vi "day 2 task 2.vi"() -> ()   [LabVIEW 2019]
panel:
  out "size(s)":i32
  out "sum":i32
  out "round scores":i32[](array[numeric])
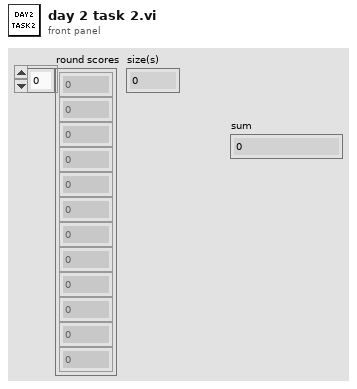
[diagram p1: front panel]
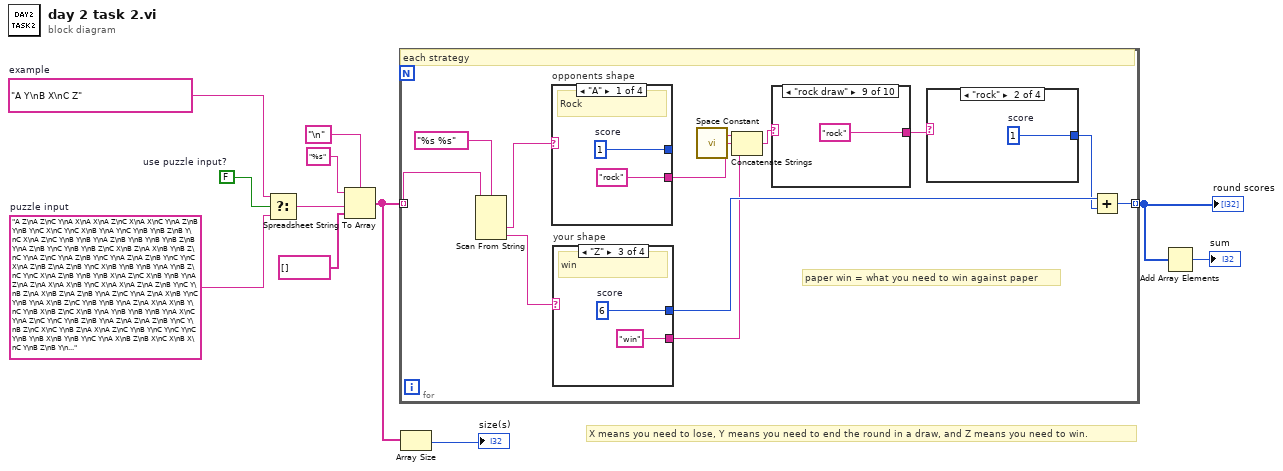
[diagram p0: block diagram]
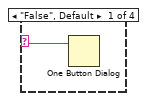
[diagram p2: hidden frame]
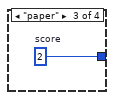
[diagram p3: hidden frame]
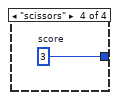
[diagram p4: hidden frame]
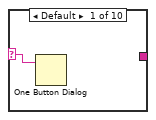
[diagram p5: hidden frame]
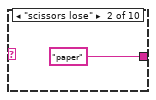
[diagram p6: hidden frame]
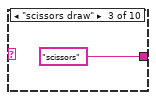
[diagram p7: hidden frame]
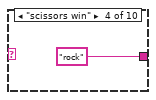
[diagram p8: hidden frame]
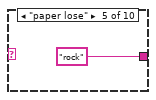
[diagram p9: hidden frame]
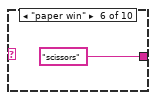
[diagram p10: hidden frame]
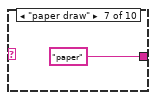
[diagram p11: hidden frame]
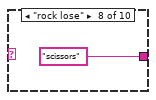
[diagram p12: hidden frame]
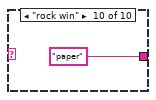
[diagram p13: hidden frame]
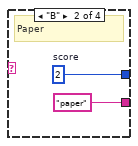
[diagram p14: hidden frame]
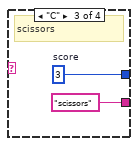
[diagram p15: hidden frame]
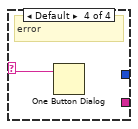
[diagram p16: hidden frame]
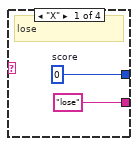
[diagram p17: hidden frame]
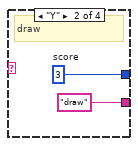
[diagram p18: hidden frame]
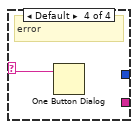
[diagram p19: hidden frame]
diagram:
  w6 = FALSE  # use puzzle input?
  w7 = "A Z\nA Z\nC Y\nA X\nA X\nA Z\nC X\nA X\nC Y\nA Z\nB Y\nB Y\nC X\nC Y\nC X\nB Y\nA Y\nC Y\nB Y\nB Z\nB Y\nC X\nA Z\nC Y\nB Y\nB Y\nA Z\nB Y\nB Y\nB Y\nB Z\nB Y\nA Z\nB Y\nC Y\nB Y\nB Z\nC X\nB Z\nA X\nB Y\nB Z\nC Y\nA Z\nC Y\nA Z\nB Y\nC Y\nA Z\nA Z\nB Y\nC Y\nC X\nA Z\nB Z\nA Z\nB Y\nC X\nB Y\nB Y\nB Y\nA Y\nB Z\nC Y\nC X\nA Z\nB Y\nB Y\nB X\nA Z\nC X\nB Y\nB Y\nA Z\nA Z\nA X\nA X\nB Y\nC X\nA X\nA Z\nA Z\nB Y\nC Y\nB Z\nA X\nB Z\nA Z\nB Y\nA Z\nC Y\nA Z\nA X\nB Y\nC Y\nB Y\nA X\nB Z\nC Y\nB Y\nB Y\nA Z\nA X\nA X\nB Y\nC Y\nB X\nB Z\nC X\nB Y\nA Y\nB Y\nB Y\nB Y\nA X\nC Y\nA Z\nC Y\nC Y\nB Z\nB Y\nA Z\nA Z\nA Z\nB Y\nC Y\nB Z\nC X\nC Y\nB Z\nA X\nA Z\nC Y\nB Y\nC Y\nC Y\nC Y\nB Y\nB X\nB Y\nB Y\nC Y\nA X\nB Z\nB X\nC X\nB X\nC Y\nB Z\nB Y\nA X\nC Y\nC Y\nC X\nB Z\nB Y\nA Y\nB Z\nA Z\nB Y\nB Y\nB Z\nB Z\nC Y\nA Z\nA X\nA X\nC Y\nB Y\nA Z\nB Z\nA X\nA Z\nB Z\nC Y\nC Z\nA X\nA Y\nB Y\nC Y\nB Y\nC Y\nB Z\nB Y\nA Z\nC Y\nB Z\nB Y\nA Z\nA Y\nB Y\nB Y\nC Y\nA Z\nC Y\nB Y\nB Y\nA X\nA Z\nA Z\nB Y\nB Y\nB Z\nC Y\nC X\nB Z\nA Y\nB Z\nA X\nC X\nA Y\nB Z\nB Z\nA X\nC X\nC X\nA Z\nC Y\nA X\nA X\nC X\nA X\nB Z\nC Z\nB Z\nB Y\nB Y\nA Z\nA Z\nB Y\nA Z\nC Y\nC X\nB Y\nA X\nA X\nB Z\nC Y\nC Y\nA X\nB Z\nA X\nC X\nC X\nB Z\nC X\nB Z\nA X\nA Y\nA X\nA Z\nA X\nB Y\nC Y\nA X\nC Y\nA Z\nB Z\nA Z\nC Y\nA X\nA Z\nB Y\nA Z\nB Z\nB Z\nA Z\nB Z\nA X\nB Y\nB Z\nC X\nB Y\nB Y\nB Y\nB Y\nA X\nB Z\nB Z\nA Z\nA Z\nC Y\nB Y\nC X\nA X\nB Y\nB Y\nC X\nB Y\nA X\nC Y\nA Z\nB Y\nA Y\nB Z\nB Y\nA Z\nA X\nB Z\nC Y\nA Z\nC Y\nC X\nB Y\nB Z\nC X\nA Y\nB Z\nA Y\nB Z\nB Z\nB Y\nB Z\nC X\nB Y\nA X\nB Z\nA Z\nB Y\nA Z\nC Y\nC Y\nC X\nC X\nA X\nC X\nA X\nA X\nB Z\nB Y\nB Y\nB Y\nB Y\nC X\nC X\nA Z\nA Z\nC X\nC X\nC Y\nC Y\nC Y\nB Y\nA Z\nC Y\nB Z\nB Z\nB Y\nC X\nC X\nC Y\nC Y\nC X\nB Z\nB Z\nB Y\nC Y\nB Y\nA Z\nC Y\nA X\nB Y\nC Y\nC Y\nC Y\nB Y\nA Z\nB Y\nA X\nB Z\nC X\nA Z\nC X\nA Z\nB Z\nC Y\nC Y\nC Y\nC X\nB Z\nC X\nB Y\nB Z\nC X\nB X\nA Z\nB Z\nB Y\nC Y\nB Z\nC Y\nA X\nB Z\nC Y\nC Y\nB Z\nB Y\nC Y\nB Z\nC Y\nA Z\nC X\nC X\nC Y\nA Z\nC Z\nC Y\nB Y\nC Y\nB Y\nB Y\nB Z\nC X\nC X\nB Z\nB Z\nB Z\nA Z\nB Y\nB Y\nA X\nB Y\nC Y\nB Y\nC X\nC X\nB Y\nB Y\nA Y\nB Z\nB Y\nB Y\nC Y\nA Z\nC X\nA Y\nB Y\nB Z\nB Y\nA Y\nC Y\nA Y\nA Z\nB Y\nA Z\nC Y\nC Y\nB Y\nA Z\nB Y\nB Y\nA Z\nB Z\nB Y\nC X\nC Y\nB Z\nB Y\nB Y\nA Z\nC Z\nA Z\nA X\nC X\nB Z\nB Z\nC X\nC Y\nB Y\nB X\nA X\nC Y\nB Z\nB Y\nC X\nB Y\nA Z\nA Z\nA X\nC Y\nB Z\nB Y\nC X\nC X\nB Y\nA Z\nC Z\nB Y\nA Z\nC Y\nB Y\nC X\nA Z\nA Z\nA X\nC X\nA X\nC X\nC X\nA Z\nC X\nB Y\nA Z\nB Y\nB Y\nC Y\nC X\nA Z\nB Z\nB Y\nB Y\nA Y\nA Z\nB Y\nA Z\nB Z\nB Y\nC Y\nA Z\nB Y\nB Y\nB Y\nC Y\nC X\nA X\nA Z\nB Z\nB Y\nC Y\nB Z\nC X\nB Y\nC X\nA Z\nB Y\nB X\nB Y\nA Y\nA X\nA X\nC X\nC X\nB Y\nB X\nC Y\nA Z\nB Z\nC Y\nC Y\nB Y\nA Z\nC X\nA Z\nC Y\nB Z\nB X\nC X\nB X\nC X\nB Y\nC Y\nC Y\nB Z\nB Y\nB Z\nB Z\nA Z\nB Y\nA Y\nB Z\nC X\nC Y\nC X\nA Z\nB Z\nC Y\nB Y\nB Z\nC X\nB Y\nA Y\nA X\nA X\nC Y\nB X\nC X\nB Z\nA Z\nA Y\nB Z\nC X\nC X\nB Y\nA X\nB Z\nC Y\nB X\nB Z\nC Y\nB Y\nC Y\nB Z\nB Y\nB Z\nB Y\nC X\nB Y\nC X\nB Z\nB Z\nC X\nB Z\nA X\nB X\nB Y\nA X\nB Z\nC X\nB Z\nB Y\nB Y\nC X\nA Y\nB Z\nB Z\nB Y\nB Y\nB Z\nC Y\nB Z\nC Y\nC X\nA Z\nC X\nA X\nC Y\nB Y\nC X\nA Z\nB Y\nA Z\nA Z\nB X\nC Y\nB Z\nC Y\nB Y\nB Z\nA X\nB Z\nA X\nC X\nB Z\nB Y\nC X\nC Y\nC Y\nB X\nC X\nC X\nB Z\nC Y\nB Z\nB Y\nB Z\nC Y\nB Y\nC Y\nC X\nB Y\nB Y\nB Z\nA Z\nC X\nA Z\nB Y\nB Z\nA Z\nC Y\nA Z\nB Y\nA Z\nA Z\nC Y\nA Y\nB Y\nA Y\nC X\nB Y\nC X\nB Z\nC Y\nA Z\nC X\nC X\nB Z\nC Z\nC Z\nB Y\nB Y\nC Y\nC Y\nA Z\nC Y\nC Y\nC Y\nA Z\nB Z\nC Y\nB Y\nC Y\nC X\nC X\nB X\nB Y\nC Y\nA Y\nB Y\nB Z\nB Y\nA Y\nB Y\nB X\nC X\nC Z\nC Y\nC Y\nC Y\nB Z\nB X\nC Y\nB Z\nC X\nC Y\nA Z\nA Y\nB Y\nC X\nA Z\nB Y\nC Y\nB Z\nA Z\nA Z\nB Y\nA Z\nC Y\nA X\nC Y\nB Z\nB Z\nB Z\nB Y\nB Y\nA Z\nA Z\nB Y\nC X\nA Z\nC Y\nB Y\nA Z\nC Y\nA Z\nB Z\nB Z\nA Y\nB Y\nB Y\nB Z\nC Z\nB Y\nB X\nB Y\nC X\nB Z\nC Y\nB Z\nA Y\nB Z\nA Z\nA X\nA Z\nC X\nC X\nB Y\nC X\nC Y\nA Z\nB Z\nB Y\nA Z\nB Z\nB Z\nB Z\nC Y\nB Y\nA X\nC Y\nC Y\nC X\nA X\nC Y\nB Y\nC X\nB Z\nA Y\nB X\nB Y\nA Z\nB Y\nB Y\nB Y\nB Z\nC X\nB Z\nB Z\nC X\nB Y\nA Y\nB Y\nC Y\nA Z\nC Z\nB Y\nB Z\nB Z\nC Y\nA Z\nC Y\nC X\nC Y\nB Y\nA X\nA X\nB Z\nC Y\nB Z\nB Y\nA Y\nC X\nA Z\nB Z\nC Y\nC Z\nC X\nB Y\nC X\nA Y\nA Y\nB Z\nC X\nB X\nC X\nB Y\nB Z\nB Z\nB Y\nC Y\nB Y\nB Y\nA Z\nB Z\nB Y\nC X\nB Z\nB Y\nB Y\nC Y\nC Z\nC X\nB Y\nA X\nC Y\nC X\nB Z\nC Y\nA X\nB Y\nA Y\nB Y\nC X\nC Y\nC X\nA X\nB Z\nC X\nB Y\nA Z\nC X\nB Y\nA Z\nB Y\nB Y\nB Y\nA Z\nA X\nC X\nC Y\nC Y\nB Y\nB Y\nB Z\nA Y\nC X\nC X\nB Y\nB Y\nB Z\nA X\nC X\nC X\nB X\nA X\nB Z\nB Y\nC X\nA X\nB Y\nC Y\nA X\nB Y\nC X\nB Z\nC Z\nB X\nC Y\nB Y\nC Y\nA Z\nC Y\nB Z\nC X\nB Z\nC X\nC Y\nC X\nC Y\nC Z\nC X\nC X\nB Y\nC Y\nC X\nC X\nB Z\nB Z\nA X\nC Y\nC Z\nB Y\nC Z\nC Y\nC X\nC X\nB Y\nC Y\nA Y\nB Y\nA Y\nB Y\nB Y\nB Y\nC Y\nC Z\nB Y\nC X\nC X\nB Z\nB Y\nB Z\nC Y\nB Z\nC X\nB Z\nB Y\nB Y\nA Z\nA X\nB X\nA X\nC X\nC Y\nB Y\nA X\nB Z\nB Y\nB Y\nA X\nC X\nC X\nB Y\nB Y\nC Y\nC Y\nB Z\nB Y\nB Y\nB Y\nC Y\nA X\nB Y\nC Y\nB Z\nB Y\nB Y\nB Z\nB Y\nB Y\nB Z\nB Y\nB Y\nC Y\nA Z\nB Z\nA Y\nB Y\nC Y\nB Z\nB Y\nB Y\nC X\nA X\nC Z\nC X\nB Y\nB Z\nC Y\nC X\nB Z\nA Z\nA Z\nC Y\nA Z\nB Y\nB Y\nB Z\nB Y\nC Y\nB Z\nC Y\nB Z\nB Z\nB Y\nC X\nB Y\nB Z\nA X\nC X\nC X\nB Z\nB Z\nC X\nB Y\nA Z\nB Y\nB Z\nC Y\nB Y\nA Z\nB Z\nB Y\nB Y\nB Y\nC X\nC Y\nA Z\nB Y\nB Y\nA Z\nA Z\nA Z\nA X\nB X\nA Z\nC Y\nC X\nA X\nB Z\nA X\nC X\nB Z\nB Y\nB Y\nC X\nA Z\nC Y\nC X\nA Y\nC X\nA Z\nB Z\nB Z\nB Y\nC Y\nB Z\nA Z\nA Z\nC Y\nB Y\nB Z\nA Z\nA Z\nB Z\nB Y\nA Z\nC Y\nA Z\nA Z\nB Y\nB Z\nB Z\nA X\nA X\nB Y\nB Z\nB Z\nC X\nB Z\nC Z\nB Y\nB Y\nB Y\nB Z\nA X\nA Z\nB Y\nA X\nB Y\nB Y\nC X\nC X\nC Y\nC Y\nA Z\nA X\nB Y\nA Z\nB Z\nB Y\nC X\nB Y\nB X\nC X\nA X\nA Z\nC Y\nC X\nC Y\nB Y\nB Y\nA X\nA Y\nB Y\nA Y\nC Y\nC X\nB Y\nB Y\nB Z\nC X\nC X\nB Y\nC X\nB Z\nC Y\nA X\nA Z\nA Z\nB Y\nA Y\nC Y\nC X\nC Y\nC Y\nB Y\nB Y\nA Z\nC X\nA X\nB Y\nB Y\nB Y\nB Z\nA Z\nB Y\nB Y\nA Z\nB Y\nA Z\nC X\nB Z\nC Y\nB Y\nB Y\nA X\nB Y\nA X\nB Y\nB Z\nC X\nB Z\nB Y\nC X\nC Y\nC Y\nA X\nA X\nB Z\nB Z\nB Y\nC X\nA Z\nC Y\nC Y\nC Y\nB Z\nB Z\nB Y\nA Z\nC Y\nA X\nA Z\nC Y\nB Z\nB Y\nB Y\nA Z\nB Y\nA Z\nC X\nA X\nB Z\nB Y\nB Y\nB Z\nA Z\nC X\nB Y\nC X\nB Z\nC X\nA Z\nB Y\nA Z\nA Z\nB Y\nC Y\nC X\nC Y\nA X\nC Y\nB Y\nB Z\nC X\nC Y\nA X\nB Z\nB Y\nC Y\nA X\nB Z\nA Y\nB Z\nB Y\nB Z\nA X\nA Z\nA X\nB Z\nC Y\nB Y\nA Y\nB Z\nA Z\nC Y\nC X\nB Z\nB Y\nC Y\nB Z\nC X\nC Y\nA X\nB Z\nB Z\nB Z\nB Z\nB Y\nC X\nB Y\nC X\nA Z\nA Z\nC Y\nA Y\nB Y\nC X\nA Z\nB Z\nC X\nC X\nA X\nB Y\nC X\nA Z\nB Y\nB Y\nB Y\nB Y\nC X\nC Y\nC Y\nB Y\nA Z\nB Y\nB Z\nB Z\nB Y\nA X\nB Z\nB Z\nC X\nC X\nC Y\nB Y\nC Y\nB Y\nB Y\nB Z\nB X\nC X\nC Y\nA Z\nB Z\nB Y\nA X\nB Z\nA Z\nB Z\nB Y\nB Y\nA Z\nC Y\nB Y\nC Y\nB Z\nB Y\nC X\nB Z\nB Z\nC Y\nC Y\nB Y\nC Y\nC X\nB X\nB Y\nC Y\nB Y\nB X\nC X\nB Y\nA Y\nA Z\nA Y\nB Z\nA Z\nA Z\nA Z\nB Y\nA Z\nA Z\nC Y\nB Z\nA Z\nA X\nB Y\nC Y\nC X\nC X\nA Z\nB Z\nB X\nB Z\nC X\nB Z\nC Y\nC X\nC Z\nC X\nB Z\nB Z\nB Z\nB Z\nA Z\nA Z\nC Y\nC Z\nC Y\nA X\nB Y\nB Y\nB Y\nA Z\nA Z\nB Z\nC Y\nC X\nB Y\nC X\nB Z\nB Y\nB Y\nB Y\nB Y\nB Y\nB X\nA Z\nA X\nA Y\nC X\nB Z\nB Y\nB Z\nC Y\nA Z\nB Z\nB Z\nC Y\nB Z\nB Z\nC X\nB Y\nC X\nB Z\nC X\nC Y\nC Y\nC X\nA Z\nA Z\nB Z\nB Y\nC X\nC X\nA Y\nA Z\nC X\nA X\nA X\nA Z\nC Y\nB Z\nB Y\nA Z\nB Y\nB Y\nB Z\nB Y\nC Y\nB Z\nA X\nB Y\nA X\nB Z\nA Z\nC X\nA X\nC Z\nA Z\nC Y\nA X\nB Y\nB Z\nB Z\nA X\nC Y\nA Z\nC X\nA Y\nC X\nB Y\nB Z\nA X\nB Y\nB Y\nA Y\nA X\nB Y\nC X\nA Y\nB Y\nB Y\nC Y\nA Z\nB Z\nA Z\nB Y\nA Z\nC Y\nC X\nB Z\nB Y\nB Z\nA X\nC Y\nC Z\nA X\nA X\nC Y\nC Y\nA Z\nC Y\nC X\nA Y\nC Y\nB Y\nB X\nB Y\nA Z\nC X\nC X\nB Y\nA Z\nA X\nB Z\nC X\nB Y\nB Y\nC Z\nA X\nA X\nB Z\nC X\nC Y\nB Z\nC Z\nB Y\nA Y\nA Z\nA Y\nC Y\nC Y\nC Y\nB Z\nB Z\nB Y\nB Y\nB Y\nB Z\nB Z\nC X\nA X\nC X\nB Y\nB Y\nB Y\nC Y\nB Y\nB Y\nC X\nA Y\nB Z\nC X\nB Z\nB Y\nA X\nC Y\nB Y\nC Y\nB Z\nB Y\nC Y\nC Z\nC Y\nA Y\nB Z\nA X\nB Z\nA Z\nA Z\nA Z\nB Y\nA X\nC Y\nB Y\nB Y\nB Y\nC X\nB Y\nA X\nC X\nB Y\nC X\nA Z\nB Z\nB Z\nB Y\nC Y\nB Y\nA Z\nB Y\nC Y\nB Z\nC X\nB Y\nB Y\nB Z\nC X\nC Y\nB Z\nB Z\nC Y\nC X\nC X\nB Y\nB Z\nA X\nC X\nA Z\nA Y\nB Z\nB Y\nB Y\nC Y\nC X\nB Y\nB Z\nC Y\nC Y\nC X\nC X\nB Z\nA Z\nB Z\nB Y\nC X\nA X\nC X\nA Z\nC X\nB Z\nC Z\nB Y\nC Y\nB Y\nC Z\nA Z\nB Y\nC Z\nA X\nB Z\nB X\nC Y\nC X\nB Z\nA Z\nB Y\nA X\nB X\nA Z\nC Y\nA Y\nA Z\nA X\nC X\nA Y\nC X\nB X\nB Y\nC Z\nA Z\nC X\nB Y\nC X\nC X\nB X\nB Y\nA Y\nB Y\nB Y\nA Z\nB Y\nC Y\nC X\nB Y\nB Y\nB Z\nC Y\nB Z\nA Z\nA Z\nA X\nB Y\nC Y\nB Y\nC Y\nC Y\nB Z\nA X\nC Y\nB Z\nC Y\nA Y\nB Y\nB Y\nB Y\nC Y\nA Z\nA Z\nB Z\nA Z\nC Y\nC Y\nB Y\nC X\nB Y\nA Z\nB Z\nA X\nB Z\nB Y\nB Z\nA X\nA X\nC Y\nA Z\nB Z\nC Y\nB Z\nC X\nB Z\nA X\nB Z\nB Z\nC Y\nB Y\nB Y\nC Y\nB Y\nA X\nB Y\nC Y\nA Z\nB Y\nC X\nA Z\nB Z\nA Z\nB Z\nC Y\nB Y\nB Y\nB Y\nC Y\nB Y\nB Y\nA Z\nB Y\nB Z\nC X\nB Z\nC X\nC X\nA X\nB Z\nC Z\nB Z\nA Y\nC X\nC X\nA Z\nA X\nA Y\nA X\nB Y\nB Y\nC X\nC Z\nA Y\nC Y\nB Y\nB Y\nC X\nC X\nB Z\nB Z\nB Y\nC Y\nA Z\nB Y\nC X\nC X\nA X\nA X\nA Y\nB Y\nC X\nA Z\nC Z\nC Y\nC Y\nC Y\nB Y\nC Y\nA Y\nA X\nB X\nB Y\nB Y\nB Y\nB Y\nA Z\nB Z\nB Y\nB Y\nC Y\nA X\nA Z\nA Z\nA Z\nB Y\nA X\nC Y\nC Y\nB Y\nB Y\nC Y\nA Z\nC Y\nA X\nC X\nB Z\nB Y\nC X\nB Y\nA X\nA Z\nC X\nC Y\nC Y\nC X\nC X\nB Z\nB Y\nA Z\nB Y\nB Z\nB Z\nB Y\nB Y\nA X\nC X\nC Y\nC X\nA Z\nB Z\nB Y\nB Y\nC Y\nA X\nA X\nC Y\nC X\nB Z\nA Y\nB Y\nB Z\nB Y\nA X\nC Y\nB Y\nA X\nC X\nB Y\nB Y\nA Z\nA Z\nA Z\nB Y\nB Y\nC X\nB Z\nA Z\nB Z\nA Z\nC X\nB Y\nC X\nB Y\nC X\nC X\nB Y\nB Y\nA Y\nC Y\nC Y\nB Z\nC X\nB Y\nB Y\nA X\nA Z\nB Y\nC Y\nB Y\nC Y\nA X\nC Y\nC Y\nB Z\nC Y\nA X\nC X\nA Z\nC Y\nA Z\nC X\nB Z\nB Y\nB Z\nC Y\nB X\nA Z\nC Y\nC X\nB Y\nC X\nB Z\nA X\nA Z\nC X\nB Z\nC X\nB Y\nA Z\nB Y\nC Y\nB Y\nC X\nC Y\nB X\nB X\nB Y\nB Y\nB Y\nB Z\nB Y\nC X\nA Z\nA Z\nC X\nB Y\nB Y\nB Y\nA Y\nC Y\nB Z\nC X\nC Y\nA X\nC Y\nB Z\nC Y\nB Y\nB Y\nB Z\nA Z\nA Z\nB Y\nA Y\nB Z\nA X\nC Y\nB Y\nA X\nC X\nB Y\nC Y\nB Z\nB Y\nC X\nA Z\nC Y\nA Z\nB Y\nC Y\nB Y\nC X\nA Z\nC Y\nC Y\nA Y\nB Z\nC X\nC X\nA Z\nC Z\nC X\nB Y\nC X\nA X\nC Y\nC X\nC X\nA X\nA Y\nA X\nC X\nA X\nA X\nB X\nB Y\nC Y\nA X\nB Z\nC X\nC Y\nB Y\nB Z\nC Y\nB Z\nB Y\nC X\nA X\nB Y\nB Z\nC Y\nA Z\nC X\nC Z\nA X\nA Z\nA Z\nB Z\nA Z\nB Y\nC Y\nC Y\nB Z\nC Y\nC Y\nC Y\nC X\nA X\nB Y\nA X\nC X\nC Z\nB Y\nA Z\nB Y\nC Y\nC Y\nB Z\nC Y\nC X\nB Z\nC Y\nB Y\nB Z\nA Z\nB Z\nB Z\nB Y\nA Z\nA Y\nC X\nB Y\nA Z\nC Y\nB Z\nA Z\nB Y\nB Y\nC Y\nB Y\nB Y\nB Y\nC Y\nB X\nB Y\nA X\nA X\nB Z\nA X\nC Y\nA Z\nB Y\nB Y\nB Z\nA Z\nC Y\nC X\nB Y\nA Z\nA X\nB Y\nC X\nB Z\nA X\nC X\nB Z\nB Z\nB Z\nB X\nA X\nC Z\nC X\nC Z\nB X\nA Z\nC X\nB Y\nC X\nC Y\nC Y\nB Y\nB Z\nB Y\nC Y\nC X\nA Z\nC Y\nC Y\nC Y\nB Z\nA Z\nA Y\nC X\nC Y\nB Y\nC Y\nC Y\nB Z\nC Y\nB Y\nB Y\nC X\nB Z\nB Y\nA X\nB Y\nA Z\nB Y\nC X\nB Y\nC X\nB Y\nA Z\nC X\nB Y\nC X\nB Z\nC X\nB Y\nA X\nC X\nC X\nA X\nC Y\nA Z\nC Y\nB Z\nA Z\nA X\nC X\nA X\nC Y\nA X\nA X\nB Z\nC X\nC Y\nA Y\nB Z\nB Y\nC Y\nB Y\nA Y\nC Y\nC Y\nB Y\nB Y\nB Z\nB Z\nC X\nB Y\nC X\nA X\nA Z\nC Y\nB Z\nC Y\nB Y\nC X\nC X\nA Z\nB Z\nA Z\nC X\nB Y\nB Z\nC Y\nB Y\nA X\nA X\nB Y\nB Y\nB Y\nA X\nB Y\nB Z\nA Z\nA X\nA X\nB Z\nB Y\nA X\nB Z\nA Z\nB Y\nB Z\nB Z\nB Z\nC Y\nC Y\nA Z\nB Y\nC Y\nA Z\nC X\nB Z\nA X\nB X\nB Y\nB Y\nC Y\nC Y\nB Z\nB Y\nA Z\nB Y\nA X\nB Z\nB Y\nC Z\nB Y\nB Y\nC Y\nB Y\nB Y\nA Y\nC Y\nA Z\nA Y\nB Z\nC X\nB Z\nA X\nA Z\nA X\nC Y\nA Z\nB Y\nB Z\nB Z\nC Y\nC Y\nC Y\nB X\nB Y\nB Z\nA X\nB Y\nC Y\nA X\nA X\nB Y\nC Y\nA Y\nB Z\nB Z\nB Z\nA Z\nB Y\nC X\nA Z\nC Y\nC Y\nB Y\nC Y\nC Y\nC Y\nC Y\nB Y\nB Z\nA Z\nB X\nC Y\nC X\nC X\nC Y\nA Z\nC Y\nC X\nB Z\nB Y\nA Y\nC Z\nB Y\nB Y\nB Y\nB Y\nC Y\nB Y\nC Y\nA Z\nB Y\nC X\nC Y\nB Z\nA X\nC Y\nB Y\nB Y\nB Y\nA Z\nA X\nA X\nC X\nC Z\nB Z\nA X\nA Z\nA X\nA Y\nC Y\nC Y\nA Z\nC X\nC X\nB X\nB Y\nA X\nA Z\nA X\nC Y\nB X\nA X\nA X\nC X\nA Y\nB Z\nA Z\nB Y\nA X\nA Z\nB Y\nA Z\nC Y\nB Z\nA Z\nC Y\nC X\nB Z\nC Y\nB Y\nC X\nA Z\nB Z\nA X\nA X\nC Z\nA X\nC X\nB Y\nB Z\nA X\nA X\nC Y\nA Z\nC Y\nC X\nC Y\nB Z\nB Y\nC X\nC X\nB Z\nB Z\nC Y\nA X\nB X\nC X\nC Y\nA X\nA Z\nB Y\nC X\nA Y\nC X\nC Y\nA Z\nB Y\nB Z\nB Y\nC X\nC Y\nC X\nC X\nB Y\nC X\nC X\nB Y\nC Z\nC Y\nC Y\nB Z\nB Z\nB Y\nA X\nB Y\nA Z\nA Y\nB Y\nC Y\nB Z\nB Z\nA X\nB Y\nA X\nB Y\nA Z\nB Y\nC X\nA Z\nB Z\nC Y\nB Y\nA Y\nA X\nC X\nA X\nB Y\nB Z\nB Z\nC Y\nA X\nB Y\nB Z\nB Y\nB X\nC Z\nB Z\nC X\nC Y\nC X\nB Z\nC Y\nA X\nA X\nC X\nB Y\nB X\nB Y\nA X\nC Y\nA Z\nB Y\nB Y\nB Y\nB Z\nB Y\nC X\nA Z\nC Y\nA Z\nB Z\nC X\nC Y\nC X\nC Y\nA Y\nB Z\nB Y\nB Z\nC Y\nA X\nB Y\nA X\nC X\nB X\nC X\nA Z\nB Z\nB Z\nC Y\nB Z"  # puzzle input
  w8 = "A Y\nB X\nC Z"  # example
  # "X means you need to lose, Y means you need to end the round in a draw, and Z means you need to win."
  n1 = Select(t=w8, s=w6, f=w7) -> (s? t:f=w5:string)
  n2 = Spreadsheet String To Array(delimiter (Tab)="\n", format string="%s", spreadsheet string=w5, array type (2D Dbl)=string[] []) -> (array=w3:string[])
  n3 = for {
    tunnel: w3 -> [w22] mode=indexing
    tunnel: [w20] -> w1 mode=indexing
    # "paper win = what you need to win against paper"
    # "each strategy"
    n4 = Scan From String(format string="%s %s", input string=w22) -> (output 1=w19:string, output 2=w21:string)  [unwired: 4 in, 3 out]
    n5 = case "opponents shape" shown="\"A\"" w19 {
      selector: w19 -> [_ _ _ w44]
      tunnel: [w39 w41 w43 _] -> _
      tunnel: ["rock" "paper" "scissors" _] -> w16
      frame "A" {
        w39 = 1  # score
        # "Rock"
      }
      frame "B" {
        w41 = 2  # score
        # "Paper"
      }
      frame "C" {
        w43 = 3  # score
        # "scissors"
      }
      frame Default {
        # "error"
        n6 = One Button Dialog(message=w44) -> ()  [unwired: 1 in, 1 out]
      }
    }
    n7 = case "your shape" shown="\"Z\"" w21 {
      selector: w21 -> [_ _ _ w51]
      tunnel: [w46 w48 w50 _] -> w18
      tunnel: ["lose" "draw" "win" _] -> w15
      frame "X" {
        w46 = 0  # score
        # "lose"
      }
      frame "Y" {
        w48 = 3  # score
        # "draw"
      }
      frame "Z" {
        w50 = 6  # score
        # "win"
      }
      frame Default {
        # "error"
        n8 = One Button Dialog(message=w51) -> ()  [unwired: 1 in, 1 out]
      }
    }
    n9 = call <vilib>:"Space Constant.vi"() -> ("String"=w14:string)
    n10 = Concatenate Strings(w16, w14, w15) -> (w17:string)
    n11 = case shown="\"rock draw\"" w17 {
      selector: w17 -> [w28 _ _ _ _ _ _ _ _ _]
      tunnel: [_ "paper" "scissors" "rock" "rock" "scissors" "paper" "scissors" "rock" "paper"] -> w13
      frame Default {
        n12 = One Button Dialog(message=w28) -> ()  [unwired: 1 in, 1 out]
      }
      frame "scissors lose" {
        # "rock"
      }
      frame "scissors draw" {
        # "rock"
      }
      frame "scissors win" {
        # "rock"
      }
      frame "paper lose" {
        # "rock"
      }
      frame "paper win" {
        # "rock"
      }
      frame "paper draw" {
        # "rock"
      }
      frame "rock lose" {
        # "rock"
      }
      frame "rock draw" {
        # "rock"
      }
      frame "rock win" {
        # "rock"
      }
    }
    n13 = case shown="\"rock\"" w13 {
      selector: w13 -> [w24 _ _ _]
      tunnel: [_ w25 w26 w27] -> w12
      frame "False", Default {
        n14 = One Button Dialog(message=w24) -> ()  [unwired: 1 in, 1 out]
      }
      frame "rock" {
        w25 = 1  # score
      }
      frame "paper" {
        w26 = 2  # score
      }
      frame "scissors" {
        w27 = 3  # score
      }
    }
    n15 = Add(x=w18, y=w12) -> (x+y=w20:i32)
  }
  "round scores" <- w1
  n16 = Array Size(array=w3) -> (size(s)=→"size(s)":i32)
  n17 = Add Array Elements(numeric array=w1) -> (sum=→"sum":i32)
